vi "Powercelltodash2.vi"() -> ()   [LabVIEW 2019]
uses:
  <vilib>/Rock Robotics/Network Tables/NT Read Number.vi
panel:
  out "Timestamp":dbl
  out "Quality":dbl
  out "X":dbl
  out "Y":dbl
  out "Z":dbl
  out "Qi":dbl
  out "Qj":dbl
  out "Qk":dbl
  out "Qv":dbl
  out "Vx":dbl
  out "Vy":dbl
  out "Vz":dbl
  out "Wx":dbl
  out "Wy":dbl
  out "Wz":dbl
  out "Ax":dbl
  out "Ay":dbl
  out "Az":dbl
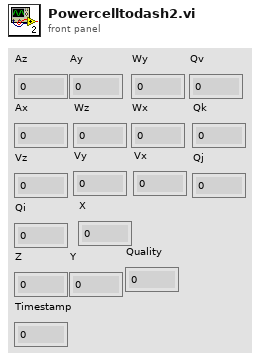
[diagram p1: front panel]
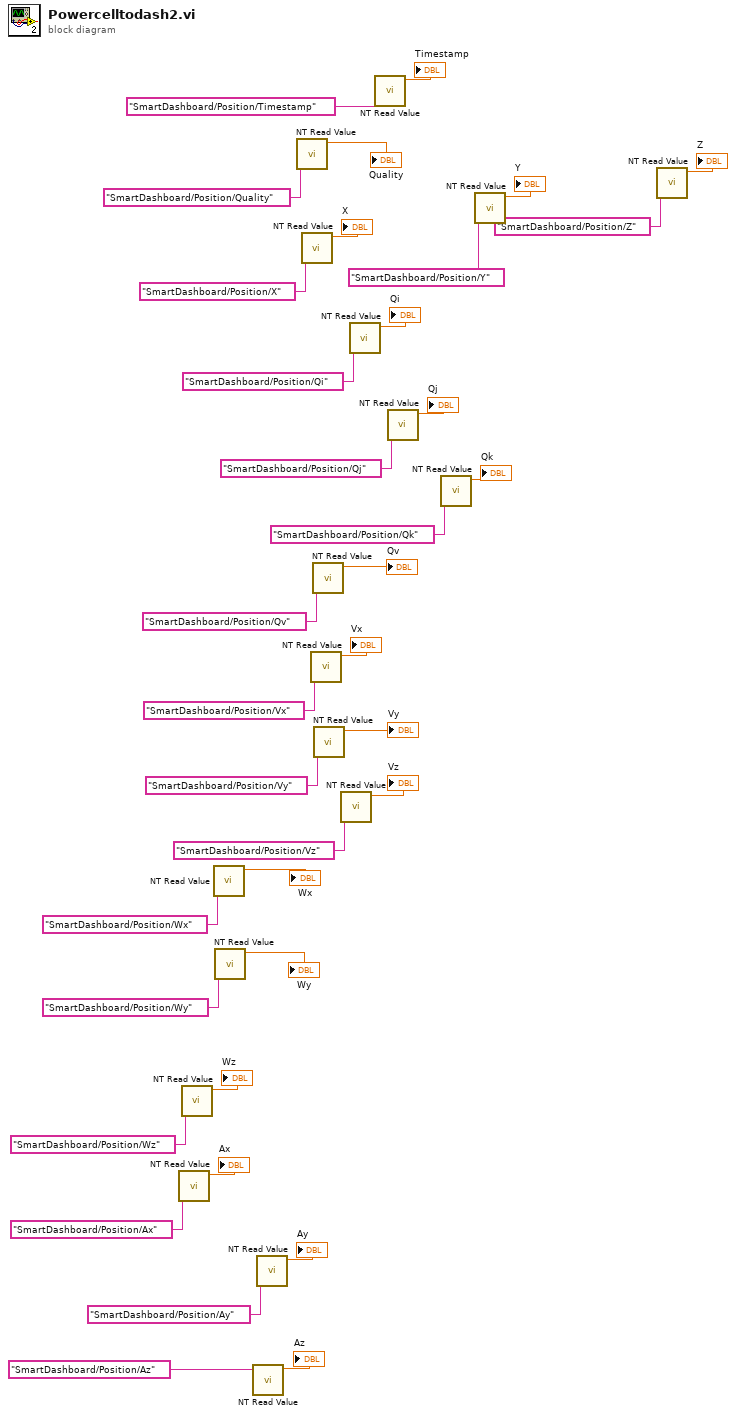
[diagram p0: block diagram]
diagram:
  n1 = call-poly <vilib>:"NT Read Value.vi"("Name"="SmartDashboard/Position/Ax") -> ("Numeric"=→"Ax":dbl)  [unwired: 9 in, 1 out]
  n2 = call-poly <vilib>:"NT Read Value.vi"("Name"="SmartDashboard/Position/Wz") -> ("Numeric"=→"Wz":dbl)  [unwired: 9 in, 1 out]
  n3 = call-poly <vilib>:"NT Read Value.vi"("Name"="SmartDashboard/Position/Wx") -> ("Numeric"=→"Wx":dbl)  [unwired: 9 in, 1 out]
  n4 = call-poly <vilib>:"NT Read Value.vi"("Name"="SmartDashboard/Position/Wy") -> ("Numeric"=→"Wy":dbl)  [unwired: 9 in, 1 out]
  n5 = call-poly <vilib>:"NT Read Value.vi"("Name"="SmartDashboard/Position/Az") -> ("Numeric"=→"Az":dbl)  [unwired: 9 in, 1 out]
  n6 = call-poly <vilib>:"NT Read Value.vi"("Name"="SmartDashboard/Position/Ay") -> ("Numeric"=→"Ay":dbl)  [unwired: 9 in, 1 out]
  n7 = call-poly <vilib>:"NT Read Value.vi"("Name"="SmartDashboard/Position/Quality") -> ("Numeric"=→"Quality":dbl)  [unwired: 9 in, 1 out]
  n8 = call-poly <vilib>:"NT Read Value.vi"("Name"="SmartDashboard/Position/X") -> ("Numeric"=→"X":dbl)  [unwired: 9 in, 1 out]
  n9 = call-poly <vilib>:"NT Read Value.vi"("Name"="SmartDashboard/Position/Vx") -> ("Numeric"=→"Vx":dbl)  [unwired: 9 in, 1 out]
  n10 = call-poly <vilib>:"NT Read Value.vi"("Name"="SmartDashboard/Position/Qv") -> ("Numeric"=→"Qv":dbl)  [unwired: 9 in, 1 out]
  n11 = call-poly <vilib>:"NT Read Value.vi"("Name"="SmartDashboard/Position/Vy") -> ("Numeric"=→"Vy":dbl)  [unwired: 9 in, 1 out]
  n12 = call-poly <vilib>:"NT Read Value.vi"("Name"="SmartDashboard/Position/Vz") -> ("Numeric"=→"Vz":dbl)  [unwired: 9 in, 1 out]
  n13 = call-poly <vilib>:"NT Read Value.vi"("Name"="SmartDashboard/Position/Qi") -> ("Numeric"=→"Qi":dbl)  [unwired: 9 in, 1 out]
  n14 = call-poly <vilib>:"NT Read Value.vi"("Name"="SmartDashboard/Position/Timestamp") -> ("Numeric"=→"Timestamp":dbl)  [unwired: 9 in, 1 out]
  n15 = call-poly <vilib>:"NT Read Value.vi"("Name"="SmartDashboard/Position/Qj") -> ("Numeric"=→"Qj":dbl)  [unwired: 9 in, 1 out]
  n16 = call-poly <vilib>:"NT Read Value.vi"("Name"="SmartDashboard/Position/Qk") -> ("Numeric"=→"Qk":dbl)  [unwired: 9 in, 1 out]
  n17 = call-poly <vilib>:"NT Read Value.vi"("Name"="SmartDashboard/Position/Y") -> ("Numeric"=→"Y":dbl)  [unwired: 9 in, 1 out]
  n18 = call-poly <vilib>:"NT Read Value.vi"("Name"="SmartDashboard/Position/Z") -> ("Numeric"=→"Z":dbl)  [unwired: 9 in, 1 out]
